vi "Pockels Cal-Scale power meter reading.vi"(11 "Power meter measured voltage (V)":dbl format="%#_13g") -> (3 "Power meter measured power (mW)":dbl)   [LabVIEW 2020]
uses:
  <vilib>/gmath/NI_Gmath.lvlib
panel:
  out "Power-meter o/p voltage (V)":dbl[](array[numeric])
  out "Power meter displayed power (mW)":dbl[](array[numeric])
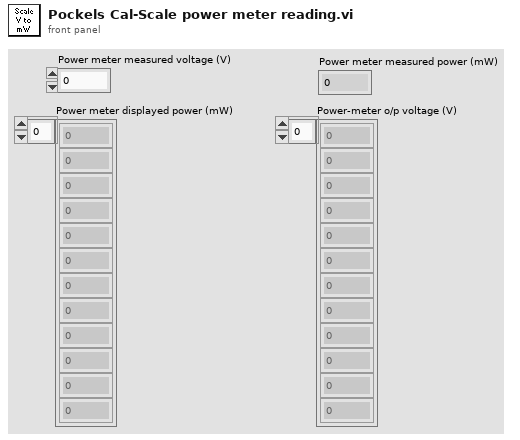
[diagram p1: front panel]
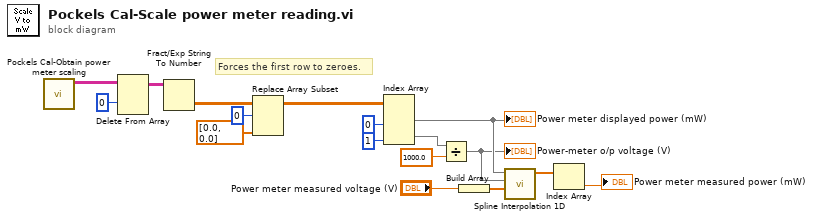
[diagram p0: block diagram]
diagram:
  # "Forces the first row to zeroes."
  n1 = call "Pockels Cal-Obtain power meter scaling.vi"() -> ("Power meter scaling/cal"=w17:string[][])  [unwired: 11 in]
  n2 = Delete From Array(array=w17, index (row)=0) -> (array with subset deleted=w15:string[][])  [unwired: 2 in, 1 out]
  n3 = Fract/Exp String To Number(string=w15) -> (number=w4:dbl[][])  [unwired: 3 in, 1 out]
  n4 = Replace Array Subset(array=w4, new element=dbl[] [0.0, 0.0] ("new element/subarray"), index (row)=0) -> (w3:dbl[][])  [unwired: 1 in]
  n5 = Index Array(array=w3, index (col) #1=0 ("disabled index (col)"), index (col) #2=1 ("index (col)")) -> (element #1=w11:dbl[], element #2=w12:dbl[])  [unwired: 2 in]
  "Power meter displayed power (mW)" <- w11
  n6 = Divide(x=w12, y=1000.0) -> (x/y=w10:dbl[])
  "Power-meter o/p voltage (V)" <- w10
  n7 = Build Array("Power meter measured voltage (V)") -> (w8:dbl[])
  n8 = call <vilib>:"Spline Interpolation 1D.vi"("xi"=w8, "X"=w10, "Y"=w11) -> ("yi"=w9:dbl[])  [unwired: 6 in, 2 out]
  n9 = Index Array(array=w9) -> (element=→"Power meter measured power (mW)":dbl)  [unwired: 1 in]
